vi "Facade.vi"(0 "Data In":T5, 2 "Display State In":T2, 3 "Container State":T4) -> (6 "Data Out":T5, 7 "Display State Out":T2, 8 "Action":T1)   [LabVIEW 2021, in "myRIO Channel Name.xctl"]
uses:
  <vilib>/myRIO/Common/Express VI Framework/xctls/myRIO Channel Name/myRIO Channel Name.xctl
  <vilib>/myRIO/Common/Express VI Framework/xctls/myRIO Channel Name/Data.ctl
  <vilib>/_xctls/Container State.ctl
  <vilib>/myRIO/Common/Express VI Framework/xctls/myRIO Channel Name/State.ctl
  <vilib>/myRIO/Common/Express VI Framework/typedefs/Data Validate Ref.ctl
  <vilib>/_xctls/Action.ctl
  <vilib>/_xctls/XControlSupport.lvlib
panel:
  in  "_Property Bundle":cluster{"Name":string, "Value":variant}[](array[cluster])
  out "Warning Icon":bool
  in  "Combo Box":string(combo)
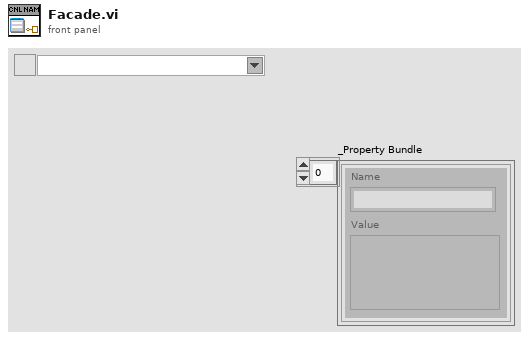
[diagram p1: front panel]
types:
  T1 = typedef "XControlSupport.lvlib/Action.ctl" = cluster{"Data Changed?":bool, "State Changed?":bool, "Action Name":string}
  T2 = typedef "myRIO Channel Name.xctl/State.ctl" = cluster{"Channel Names":string[], "Data Valid":T3, "Current Channel":string}
  T3 = typedef "Data Validate Ref.ctl" = refnum<user-event>
  T4 = typedef "XControlSupport.lvlib/Container State.ctl" = cluster{"Indicator?":bool, "Run Mode?":bool, " Refnum":refnum<vi>}
  T5 = typedef "myRIO Channel Name.xctl/Data.ctl" = u16
  T6 = cluster{"Combo Box":refnum<vi>, "Warning Icon":refnum<vi>}
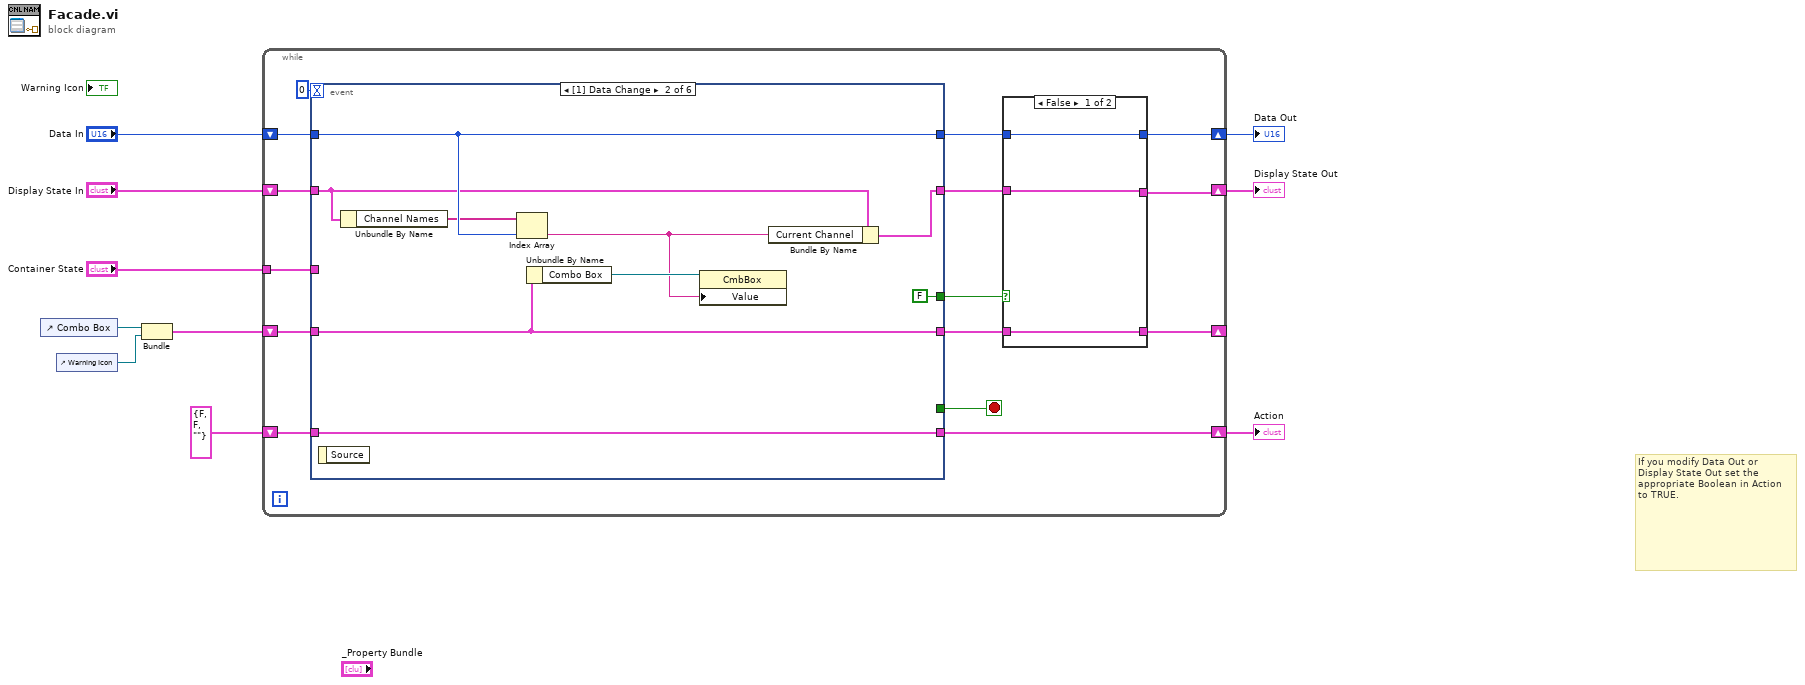
[diagram p0: block diagram]
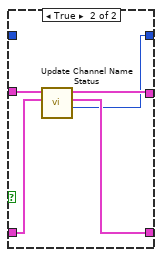
[diagram p2: hidden frame]
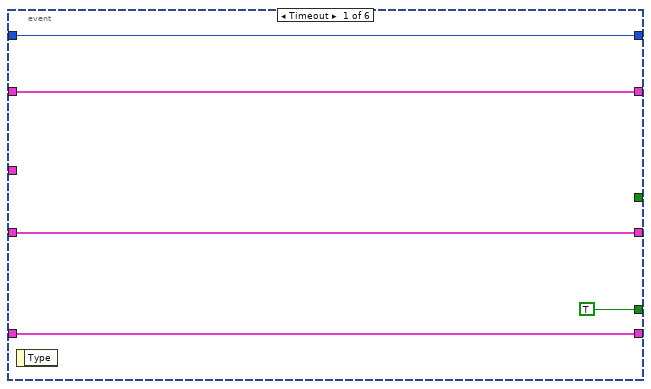
[diagram p3: hidden frame]
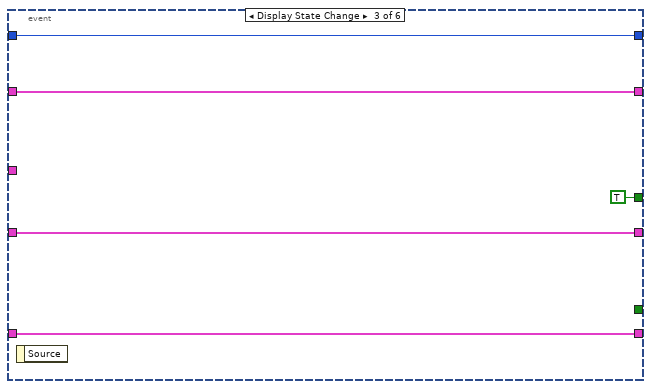
[diagram p4: hidden frame]
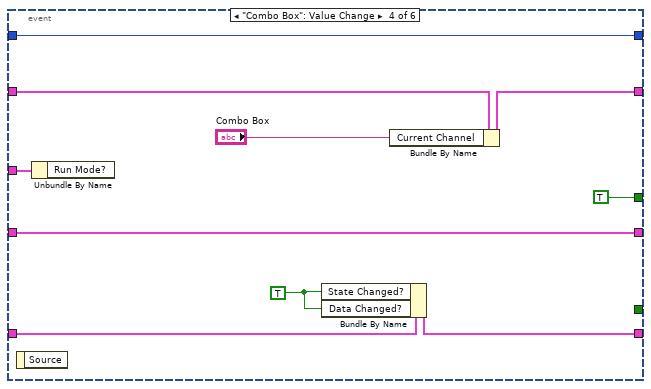
[diagram p5: hidden frame]
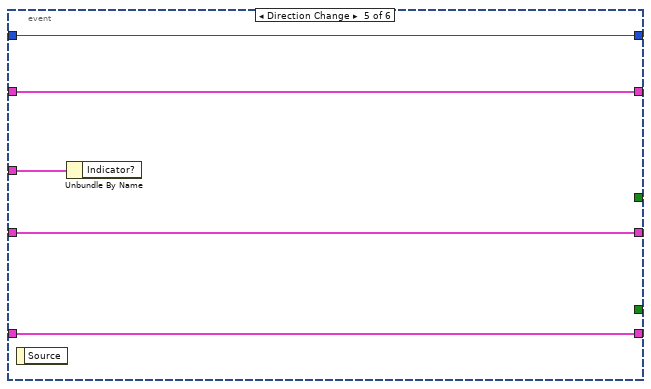
[diagram p6: hidden frame]
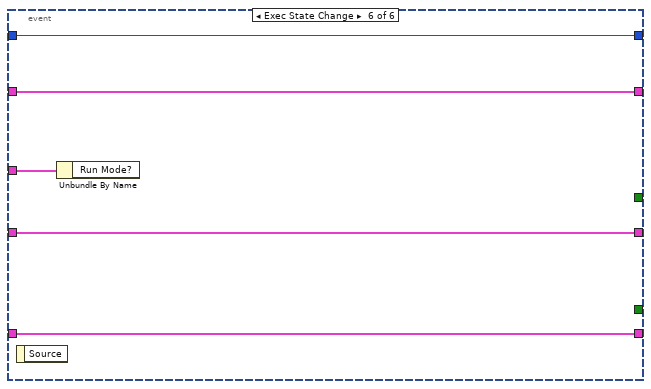
[diagram p7: hidden frame]
diagram:
  # "If you modify Data Out or\nDisplay State Out set the\nappropriate Boolean in Action\nto TRUE."
  n1 = control-ref of="Combo Box"() -> (w3:refnum<vi>)
  n2 = control-ref of="Warning Icon"() -> (w2:refnum<vi>)
  n3 = Bundle("Combo Box"=w3, "Warning Icon"=w2) -> (w1:T6)  [unwired: 1 in]
  n4 = while {
    shift-right: [w11] -> w7
    shift-left: "Display State In" -> [w25]
    tunnel: "Container State" -> [w22]
    shift-right: [w17] -> w10
    shift-left: "Data In" -> [w21]
    shift-right: [w19] -> w5
    shift-left: T1 {"Data Changed?"=FALSE, "State Changed?"=FALSE, "Action Name"=""} ("Action") -> [w20]
    shift-right: [w14] -> _
    shift-left: w1 -> [w15]
    stop <- w24 stop-if-true
    n5 = event shown="[1] Data Change" {
      selector: _ -> [_ _ _ _ _ _]
      dyn-events: _ -> [_ _ _ _ _ _]
      timeout: 0 -> [_ _ _ _ _ _]
      tunnel: w25 -> [w36 w42 w50 w62 w66 w71]
      tunnel: [w36 w40 w50 w56 w66 w71] -> w13
      tunnel: [TRUE _ _ _ _ _] -> w24
      tunnel: w22 -> [_ _ _ w54 w67 w72]
      tunnel: w21 -> [w35 w46 w48 w57 w65 w70]
      tunnel: [w35 w46 w48 w57 w65 w70] -> w16
      tunnel: [w37 w39 w52 w60 w64 w69] -> w19
      tunnel: w20 -> [w37 w39 w52 w61 w64 w69]
      tunnel: [_ FALSE TRUE TRUE _ _] -> w18
      tunnel: w15 -> [w34 w44 w49 w55 w63 w68]
      tunnel: [w34 w44 w49 w55 w63 w68] -> w12
      event Timeout {
        n6 = event-data() -> ()  [unwired: 1 in, 1 out]
      }
      event Data Change {
        n7 = event-data() -> ()  [unwired: 1 in, 1 out]
        n8 = Unbundle By Name(w42) -> ("Channel Names"=w45:string[])
        n9 = Index Array(array=w45, index=w46) -> (element=w41:string)
        n10 = Unbundle By Name(w44) -> ("Combo Box"=w43:refnum<vi>)
        n11 = property class="CmbBox"(reference=w43, "Value"=w41) -> ()  [unwired: 1 in, 2 out]
        n12 = Bundle By Name(cluster=w42, "Current Channel"=w41) -> (w40:T2)
      }
      event Display State Change {
        n13 = event-data() -> ()  [unwired: 1 in, 1 out]
      }
      event "Combo Box": Value Change {
        w53 = TRUE ("Data Changed?")
        n14 = event-data() -> ()  [unwired: 1 in, 1 out]
        n15 = Unbundle By Name(w54) -> ()  [unwired: 1 out]
        n16 = Bundle By Name(cluster=w61, "State Changed?"=w53, "Data Changed?"=w53) -> (w60:T1)
        n17 = Bundle By Name(cluster=w62, "Current Channel"="Combo Box") -> (w56:T2)
      }
      event Direction Change {
        n18 = event-data() -> ()  [unwired: 1 in, 1 out]
        n19 = Unbundle By Name(w67) -> ()  [unwired: 1 out]
      }
      event Exec State Change {
        n20 = event-data() -> ()  [unwired: 1 in, 1 out]
        n21 = Unbundle By Name(w72) -> ()  [unwired: 1 out]
      }
    }
    n22 = case shown="False" w18 {
      tunnel: [w26 w29] -> w17
      tunnel: w16 -> [w26 _]
      tunnel: [w27 w30] -> w14
      tunnel: w13 -> [w28 w33]
      tunnel: w12 -> [w27 w32]
      tunnel: [w28 w31] -> w11
      frame False {
      }
      frame True {
        n23 = call <vilib>:"Update Channel Name Status.vi"("Ctl Reference"=w32, "Display State In"=w33) -> ("Data"=w29:u16, "Ctl Reference Out"=w30:T6, "Display StateOut"=w31:T2)  [unwired: 6 in, 1 out]
      }
    }
  }
  "Display State Out" <- w7
  "Data Out" <- w10
  "Action" <- w5
